vi "convert dds config.vi"(11 "reader configuration":T2) -> (3 "writer configuration":T1)   [LabVIEW 2013, in "dds configuration.lvclass"]
uses:
  dds configuration.lvclass
  <vilib>/RTI DDS Toolkit for LabVIEW/Types/RTI DDS Advanced Reader Configuration.ctl
  <vilib>/RTI DDS Toolkit for LabVIEW/Types/RTI DDS Advanced Writer Configuration.ctl
  <vilib>/RTI DDS Toolkit for LabVIEW/Library/LVDDS_library.lvlib
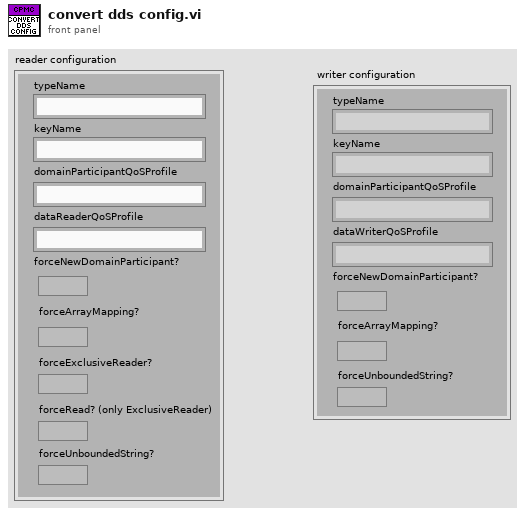
[diagram p1: front panel]
types:
  T1 = typedef "LVDDS_library.lvlib/RTI DDS Advanced Writer Configuration.ctl" = cluster{"typeName":string, "keyName":string, "domainParticipantQoSProfile":string, "dataWriterQoSProfile":string, "forceNewDomainParticipant?":bool, "forceArrayMapping?":bool, "forceUnboundedString?":bool}
  T2 = typedef "LVDDS_library.lvlib/RTI DDS Advanced Reader Configuration.ctl" = cluster{"typeName":string, "keyName":string, "domainParticipantQoSProfile":string, "dataReaderQoSProfile":string, "forceNewDomainParticipant?":bool, "forceArrayMapping?":bool, "forceExclusiveReader?":bool, "forceRead? (only ExclusiveReader)":bool, "forceUnboundedString?":bool}
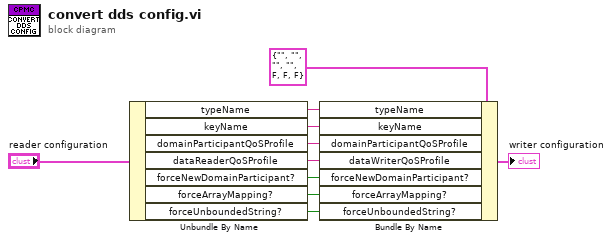
[diagram p0: block diagram]
diagram:
  n1 = Unbundle By Name("reader configuration") -> ("typeName"=w7:string, "keyName"=w6:string, "domainParticipantQoSProfile"=w5:string, "dataReaderQoSProfile"=w4:string, "forceNewDomainParticipant?"=w3:bool, "forceArrayMapping?"=w2:bool, "forceUnboundedString?"=w1:bool)
  n2 = Bundle By Name(cluster=T1 {"typeName"="", "keyName"="", "domainParticipantQoSProfile"="", "dataWriterQoSProfile"="", "forceNewDomainParticipant?"=FALSE, "forceArrayMapping?"=FALSE, "forceUnboundedString?"=FALSE} ("writer configuration"), "typeName"=w7, "keyName"=w6, "domainParticipantQoSProfile"=w5, "dataWriterQoSProfile"=w4, "forceNewDomainParticipant?"=w3, "forceArrayMapping?"=w2, "forceUnboundedString?"=w1) -> (→"writer configuration":T1)
